vi "Diameter_To_Area_Calc.vi"(8 "error in":errorcluster, 11 "Diameter (in)":dbl) -> (0 "error out":errorcluster, 3 "Area (ft^2)":dbl)   [LabVIEW 2025]
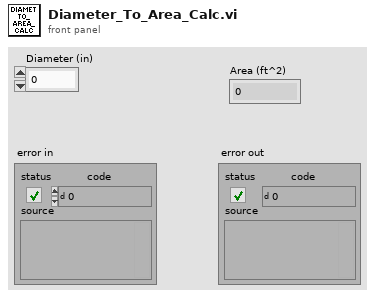
[diagram p1: front panel]
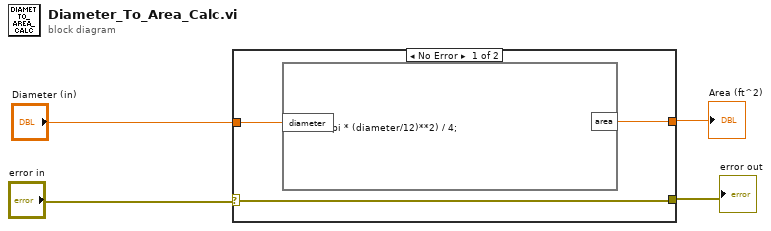
[diagram p0: block diagram]
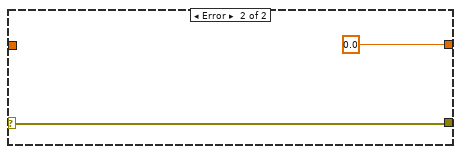
[diagram p2: hidden frame]
diagram:
  n1 = case shown="No Error" "error in" {
    selector: "error in" -> [w5 w9]
    tunnel: "Diameter (in)" -> [w7 _]
    tunnel: [w6 0.0 ("area")] -> w4
    tunnel: [w5 w9] -> w3
    frame No Error {
      n2 = formula code="area = (pi * (diameter/12)**2) / 4;"("diameter"=w7) -> ("area"=w6:dbl)
    }
    frame Error {
    }
  }
  "Area (ft^2)" <- w4
  "error out" <- w3
